vi "Override To Nominal State.vi"(11 "TEMPLATE jettl in":refnum<class "TEMPLATE Actor.lvclass">) -> (3 "TEMPLATE jettl out":refnum<class "TEMPLATE Actor.lvclass">)   [LabVIEW 2021, in "_Template.lvlib" / "Templates.lvlib" / "TEMPLATE Actor.lvlib" / "TEMPLATE Actor.lvclass"]
uses:
  TEMPLATE Actor.lvclass
  jettl/jettl/jettl/jettl.lvclass
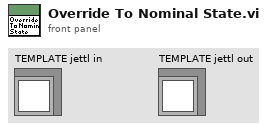
[diagram p1: front panel]
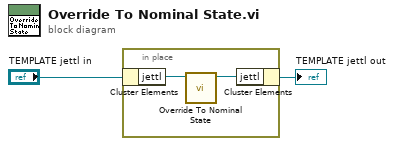
[diagram p0: block diagram]
diagram:
  n1 = in-place {
    n2 = in-place-cluster #1("TEMPLATE jettl in") -> ("jettl"=w4:refnum<class "jettl.lvclass">)
    n3 = call-dynamic "Override To Nominal State.vi"("jettl in"=w4) -> ("jettl out"=w3:refnum<class "jettl.lvclass">)  [unwired: 10 in]
    n4 = in-place-cluster #1("jettl"=w3) -> (→"TEMPLATE jettl out":refnum<class "TEMPLATE Actor.lvclass">)
  }
